vi "StartStopCounter.vi"(8 "error in (no error)":errorcluster, 10 "Start/Stop":bool, 11 "Digital Acquisition in":refnum<class "Digital Acquisition.lvclass">) -> (0 "error out":errorcluster, 3 "Digital Acquisition out":refnum<class "Digital Acquisition.lvclass">)   [LabVIEW 2020, in "Digital Acquisition.lvlib" / "Digital Acquisition.lvclass"]
uses:
  Digital Acquisition.lvclass
  Digital Acquisition.lvclass/Digital Acquisition.ctl
  Counter/Counter Messages/StartStop Msg/StartStop Msg.lvclass/StartStop Msg.ctl
  <vilib>/ActorFramework/Message Enqueuer/Message Enqueuer.lvclass/Message Enqueuer.ctl
  <vilib>/ActorFramework/Message Enqueuer/Enqueue.vi
  Counter/Counter Messages/StartStop Msg/StartStop Msg.lvclass
  C:/Program Files (x86)/National Instruments/LabVIEW 2020/vi.lib/ActorFramework/Message/Message.lvclass
  <vilib>/ActorFramework/Message Priority Queue/Priority Enqueue.vi
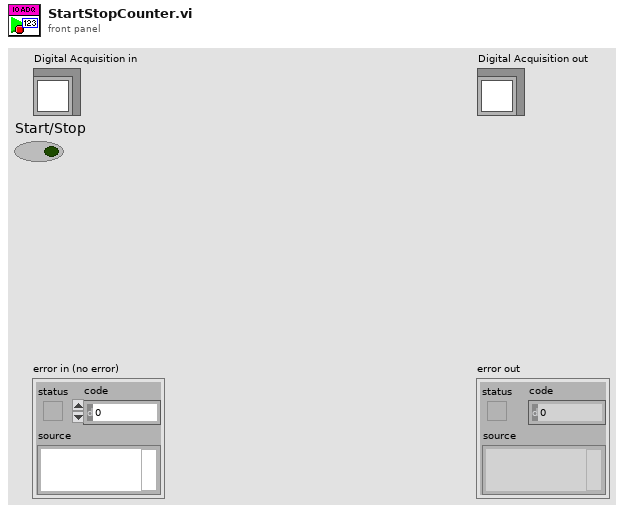
[diagram p1: front panel]
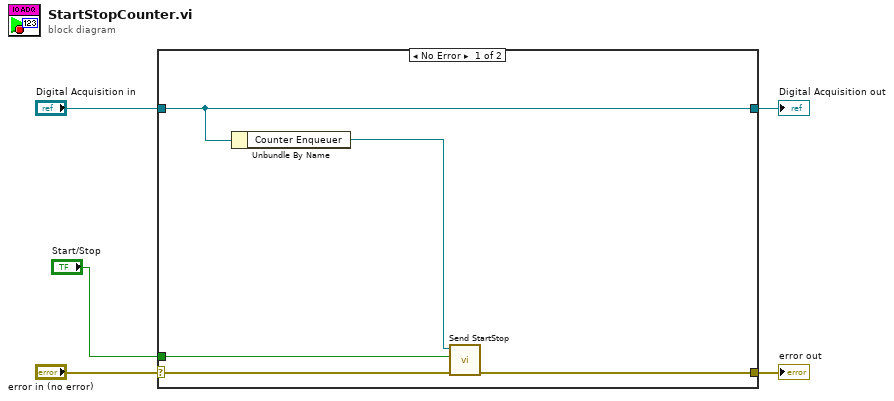
[diagram p0: block diagram]
diagram:
  n1 = case shown="No Error" "error in (no error)" {
    selector: "error in (no error)" -> [w9 w12]
    tunnel: [w8 w12] -> w4
    tunnel: [w10 w11] -> w2
    tunnel: "Digital Acquisition in" -> [w10 w11]
    tunnel: "Start/Stop" -> [w6 _]
    frame No Error {
      n2 = Unbundle By Name(w10) -> ("Counter Enqueuer"=w7:refnum<class "Message Enqueuer.lvclass">)
      n3 = call "Send StartStop.vi"("error in (no error)"=w9, "Start/Stop"=w6, "Message Enqueuer"=w7) -> ("error out"=w8:errorcluster)  [unwired: 7 in, 1 out]
    }
    frame Error {
    }
  }
  "error out" <- w4
  "Digital Acquisition out" <- w2
